vi "VG_progressBar.vi"() -> ()   [LabVIEW 2020]
panel:
  out "progression":dbl(slide) scale=0.0..100.0
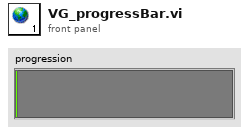
[diagram p1: front panel]
diagram:
